vi "ResultsDB Select data_FGV.vi"(6 "Upload Num":string="1", 7 "CMD":T1(ring), 8 "error in (no error)":errorcluster, 9 "ItemsID":string, 11 "MainBarcode":string) -> (0 "error out":errorcluster, 2 "File Paht":string[](array[string]), 3 "30 rows":string[][](array[string]))   [LabVIEW 2021, in "SQLite.lvclass"]
doc: "开始测试时根据条目自动创建条目条目，生产文件路径。\n#2020-6-8 13:25:45"
uses:
  SQLite.lvclass
  <vilib>/Utility/error.llb/Trim Whitespace.vi
  SQLite.lvclass/SQLite.ctl
  <userlib>/LabSQL/LabSQL.lvlib
  vi.lib_New/TopPath/TopPath.lvlib
  <userlib>/sushu/sushu.lvlib
panel:
  in  "error in (no error) 2":errorcluster
  out "32bit integer":i32
  out "size(s)":i32
  out "Update CMD":string
  out "element":string
  out "Table Control":string[][](table)
  out "CMD":string
  out "error out 2":errorcluster
  out "match substring":string
  out "number (0 to 1)":dbl
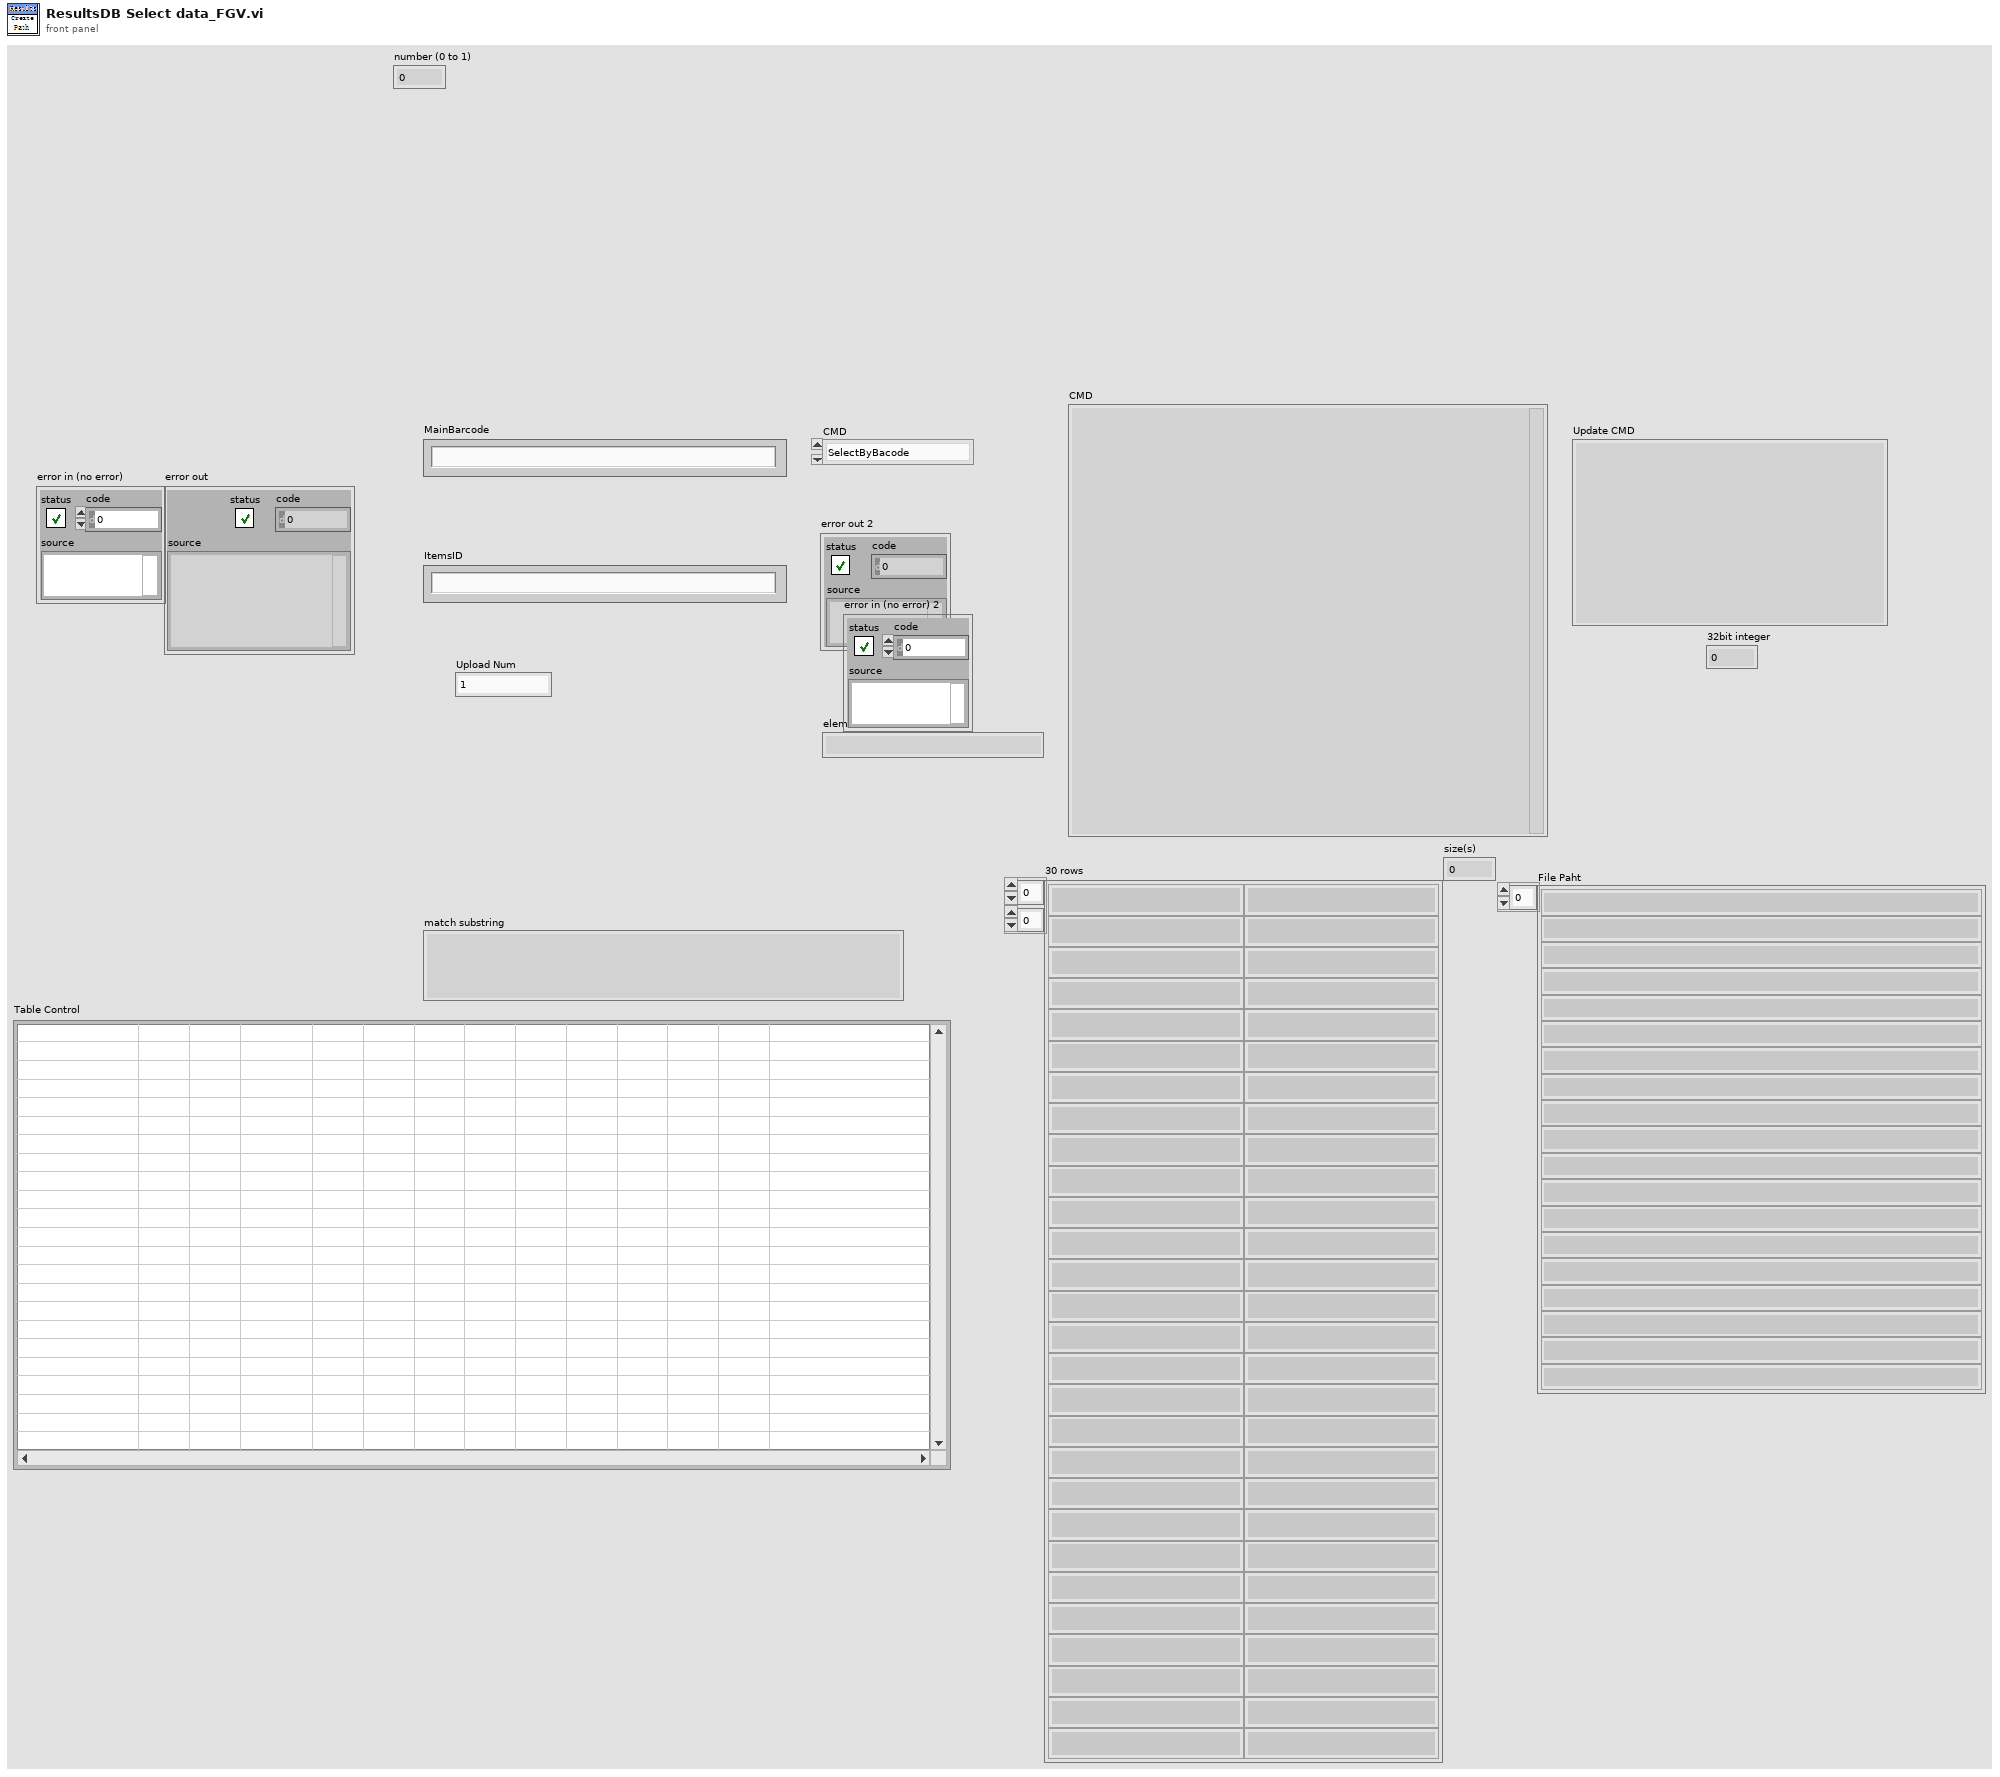
[diagram p1: front panel]
types:
  T1 = enum16{"SelectByBacode", "SelectByDatetime", "Update-UploadColumn"}
  T2 = cluster{"Core":cluster{"Current VI Reference":refnum<vi>, "Close Panel on Exit?":bool}, "VI Name":string, "Row Numbers":string, "Update?":bool, "Results Folder path":path, "CMD":string, "RowNum":i32, "ResultFilePath":path, "InsertTimes":i32, "length":i32}
  T3 = typedef "TopPath.lvlib/Top Path.ctl" = cluster{"LV Source":path, "FilePath":path, "Data":path}
  T4 = enum16{"Other", "SQL2008", "SQLite", "Access", "MySQL"}
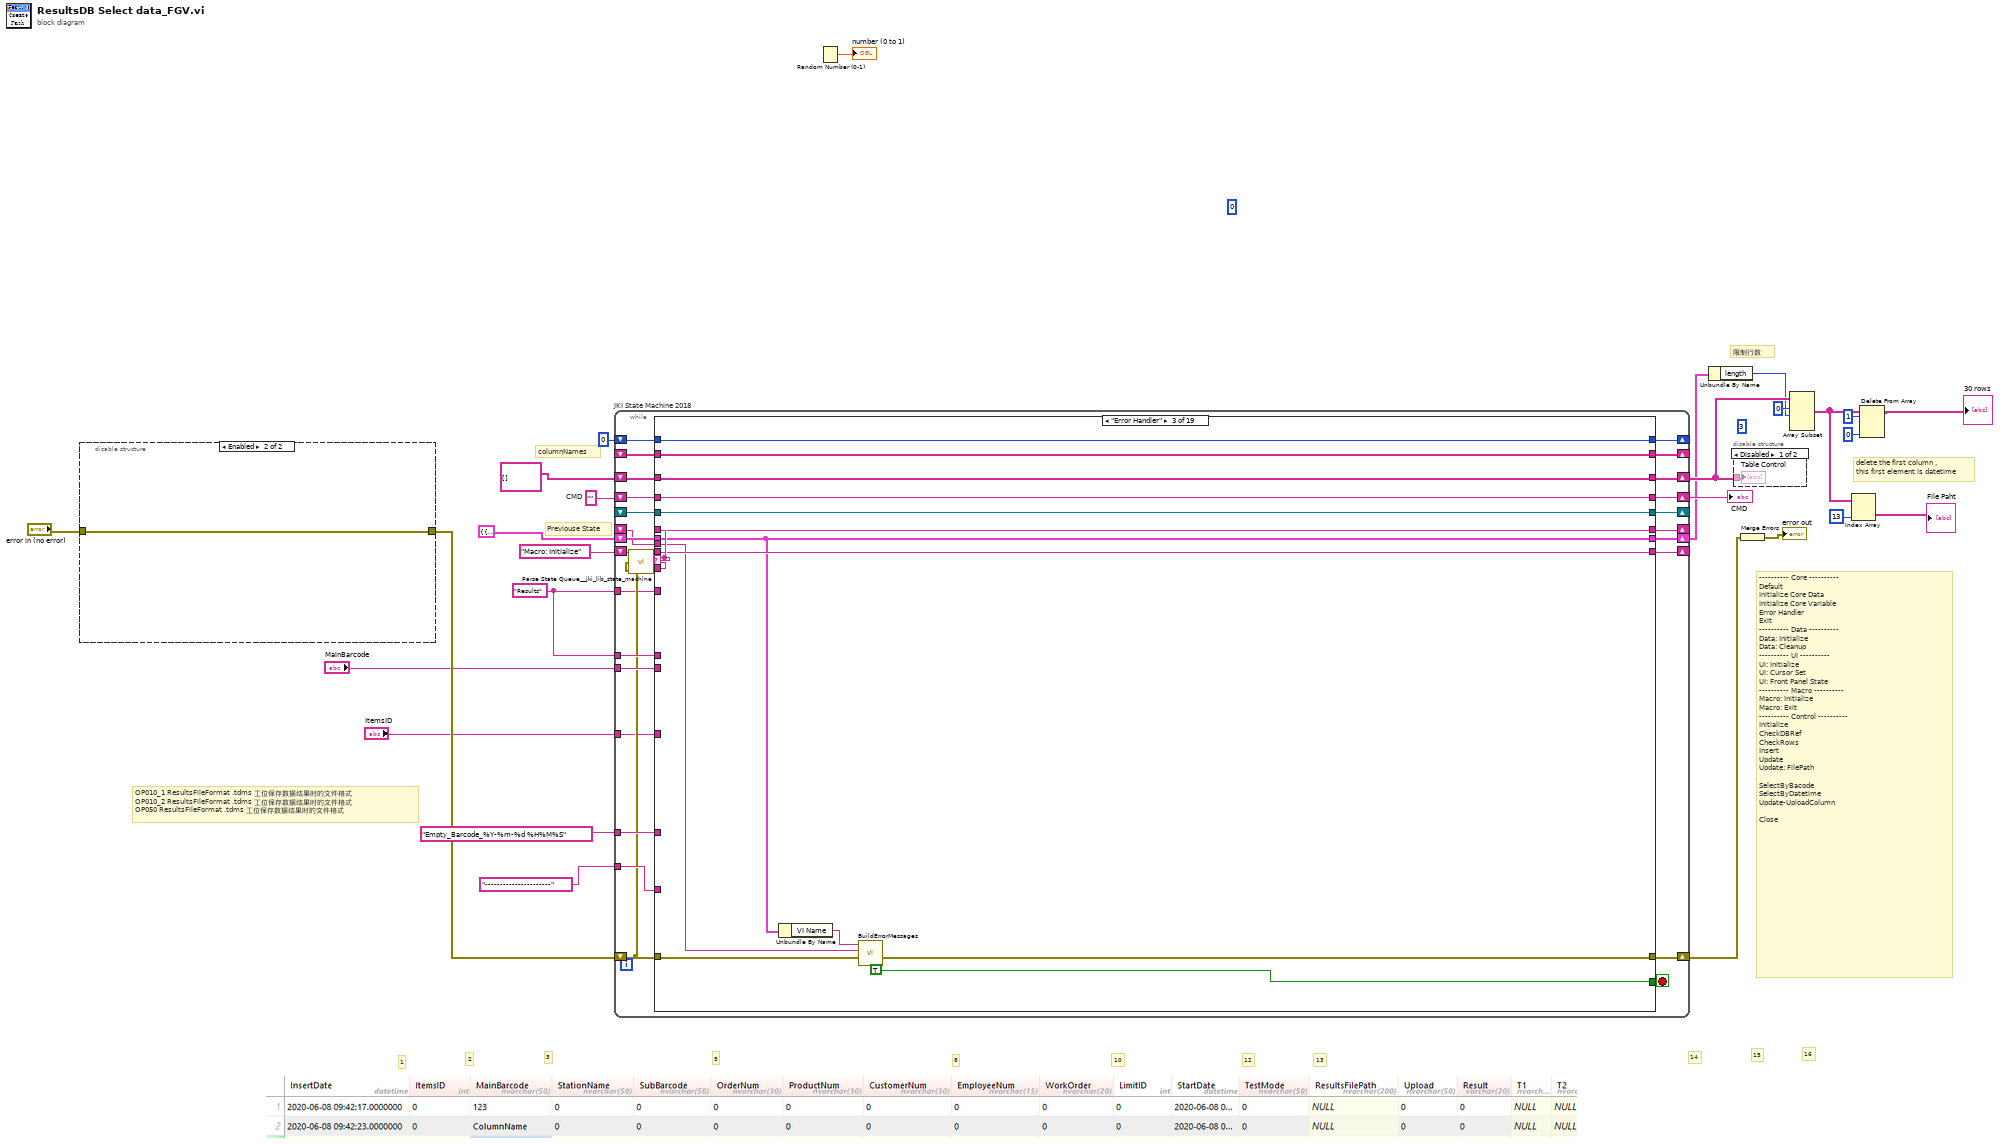
[diagram p0: block diagram]
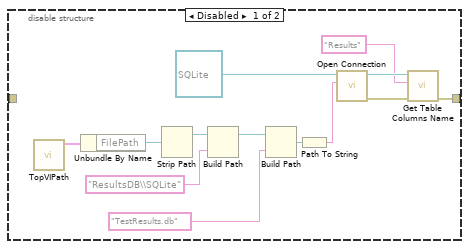
[diagram p2: hidden frame]
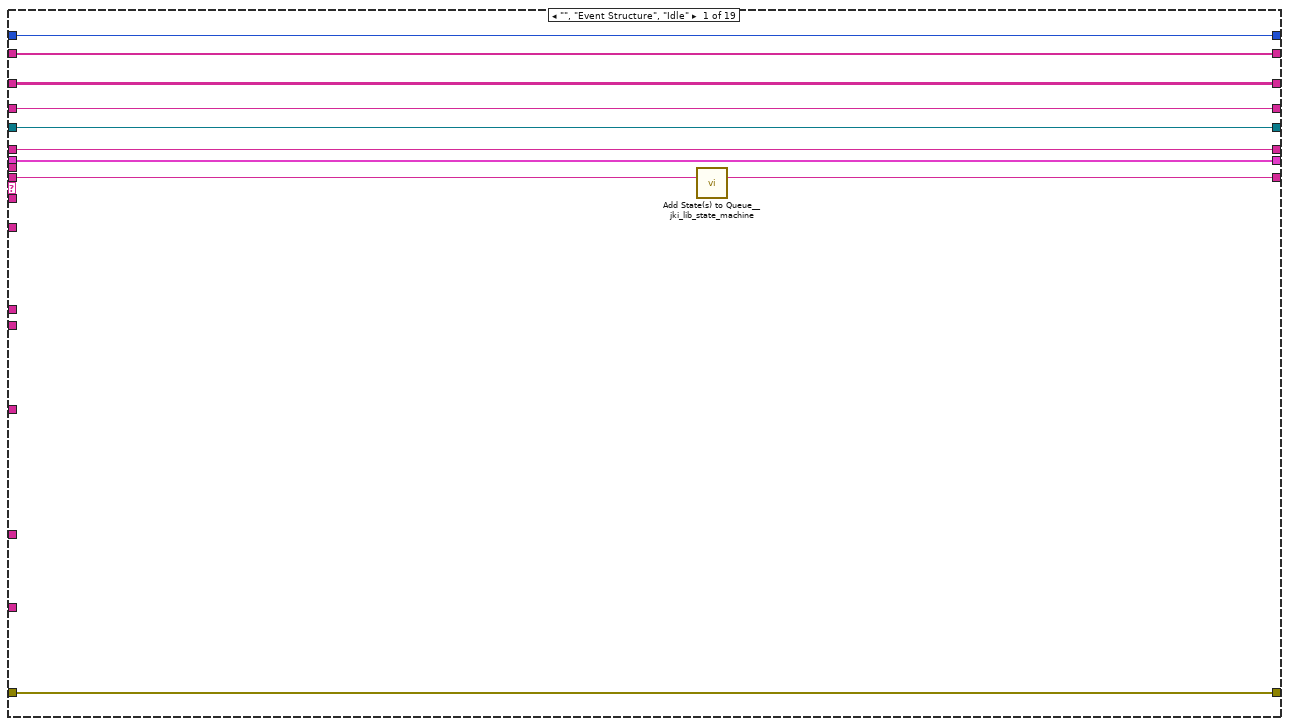
[diagram p4: hidden frame]
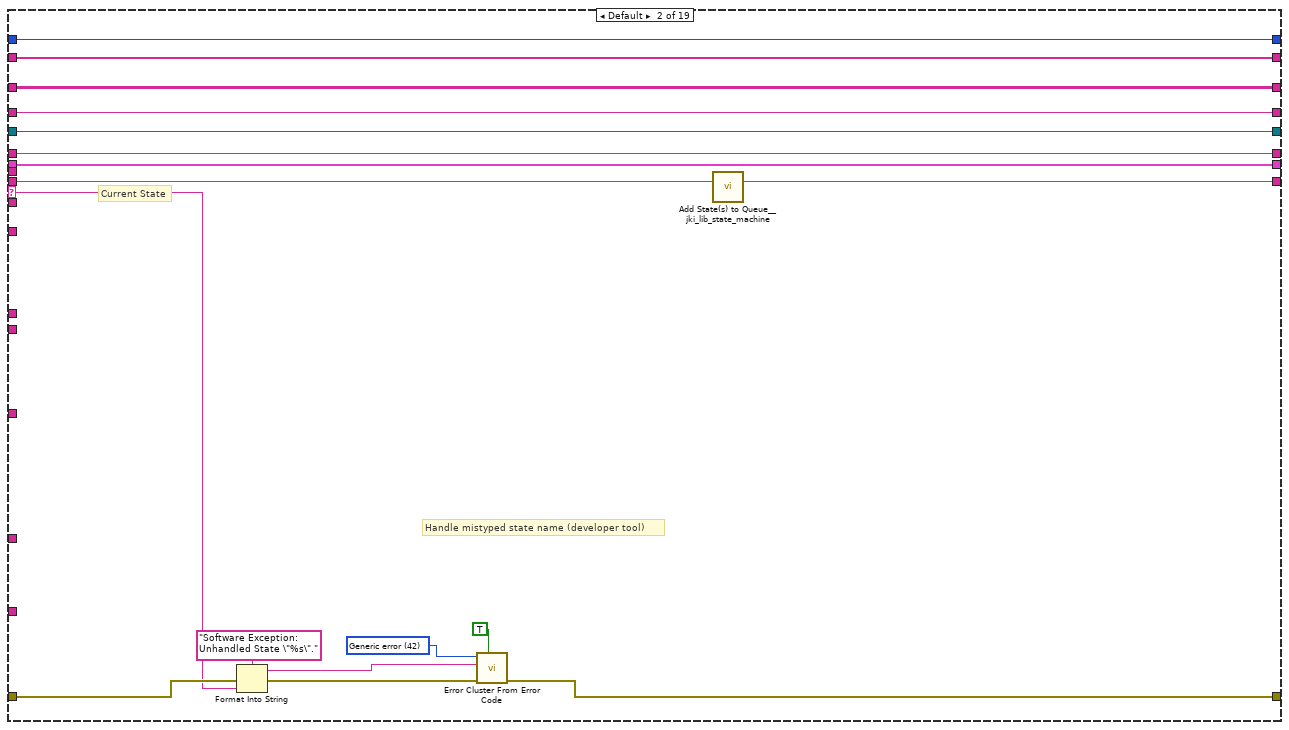
[diagram p5: hidden frame]
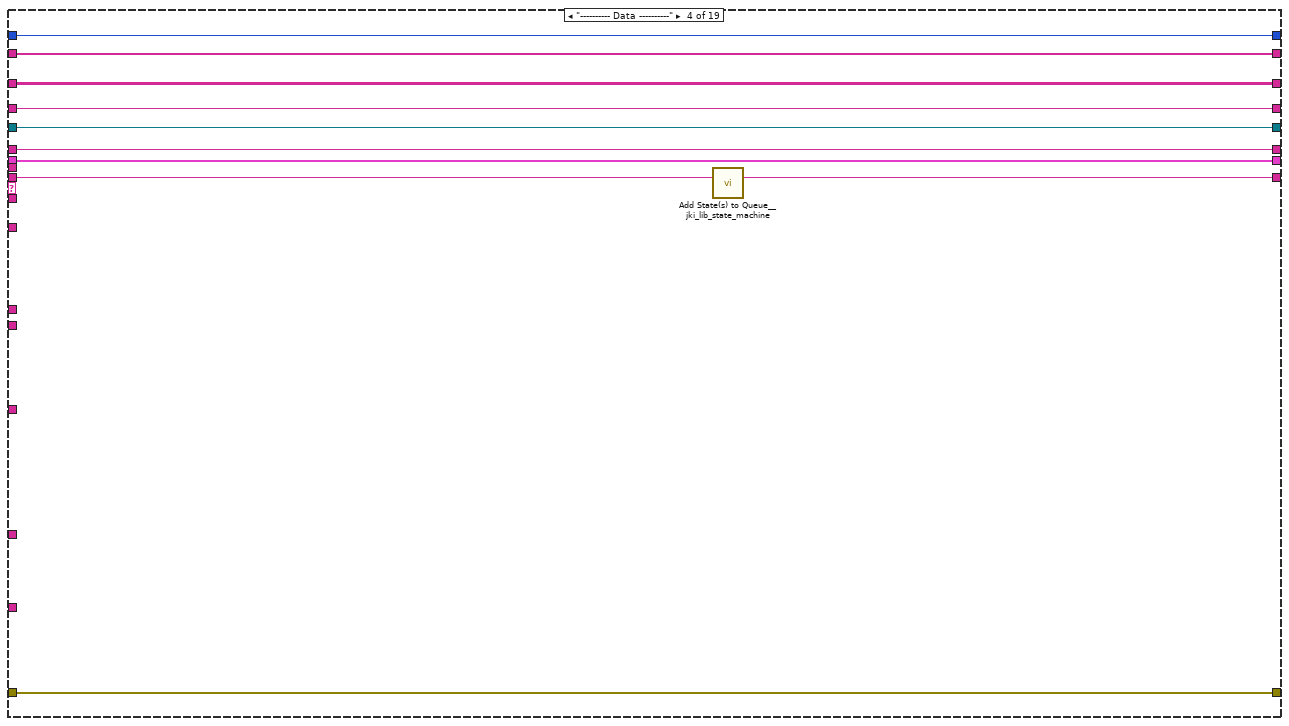
[diagram p6: hidden frame]
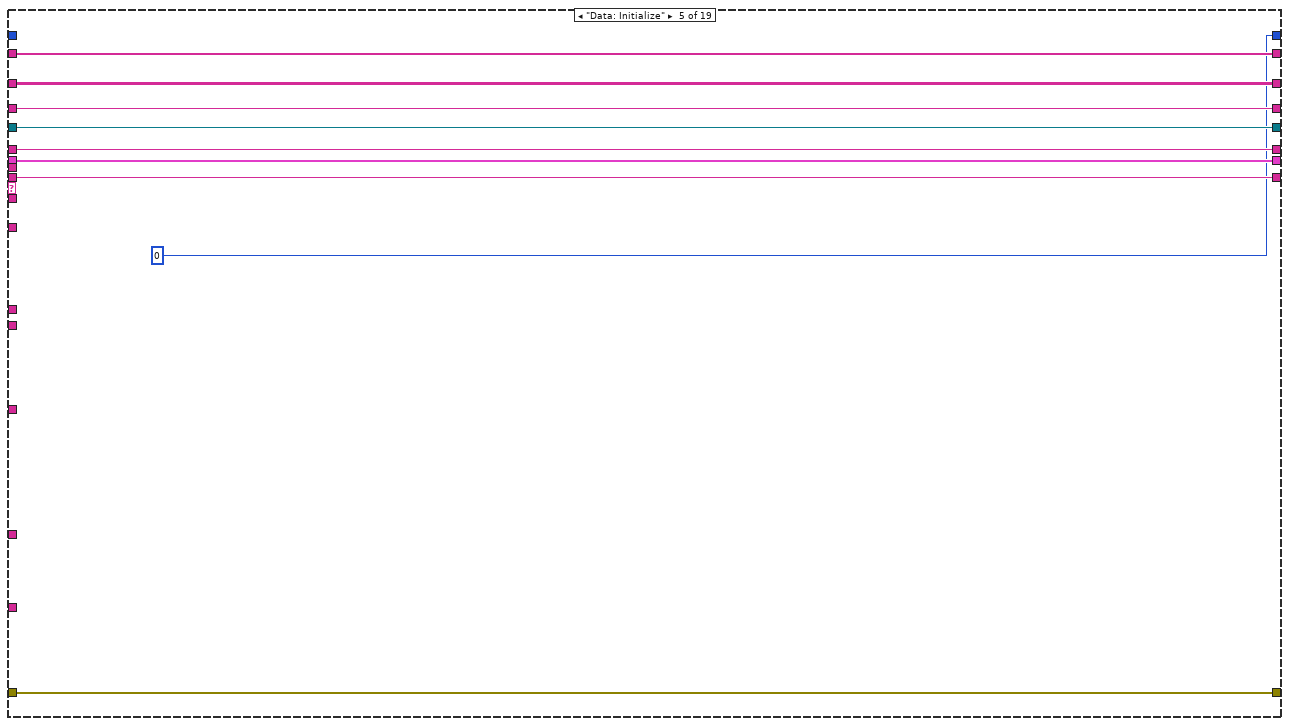
[diagram p7: hidden frame]
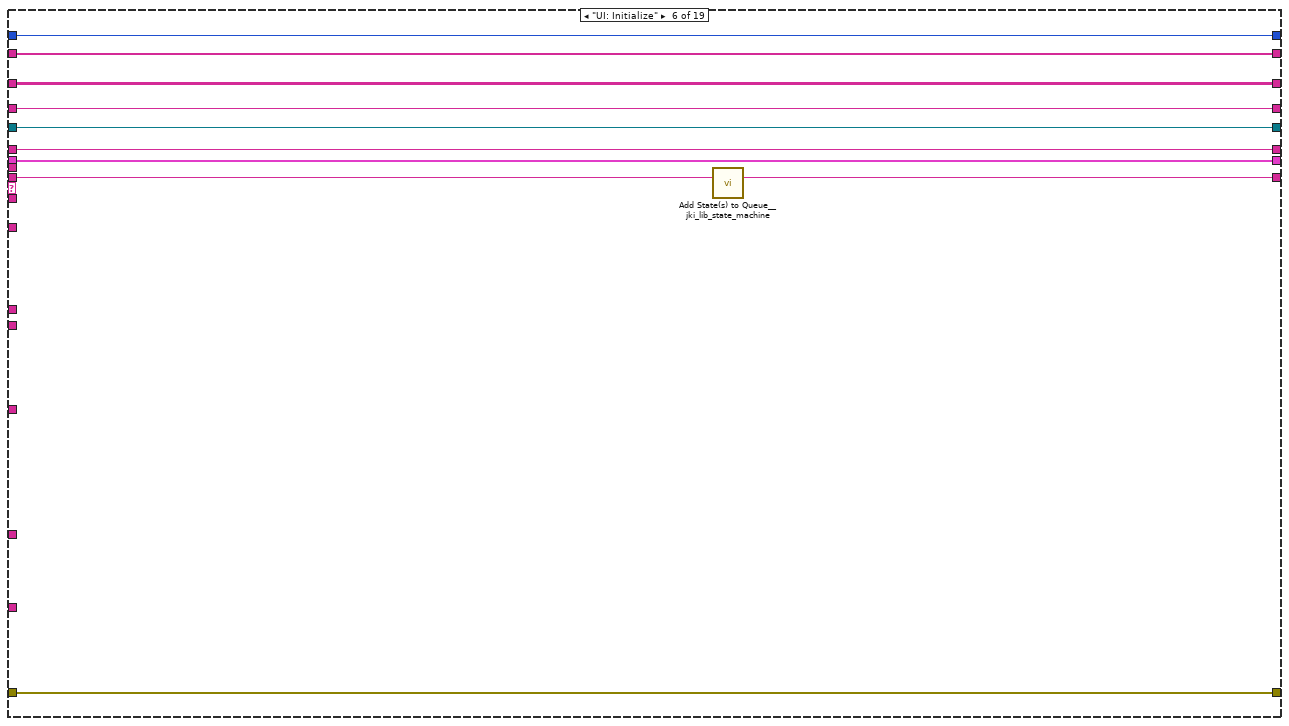
[diagram p8: hidden frame]
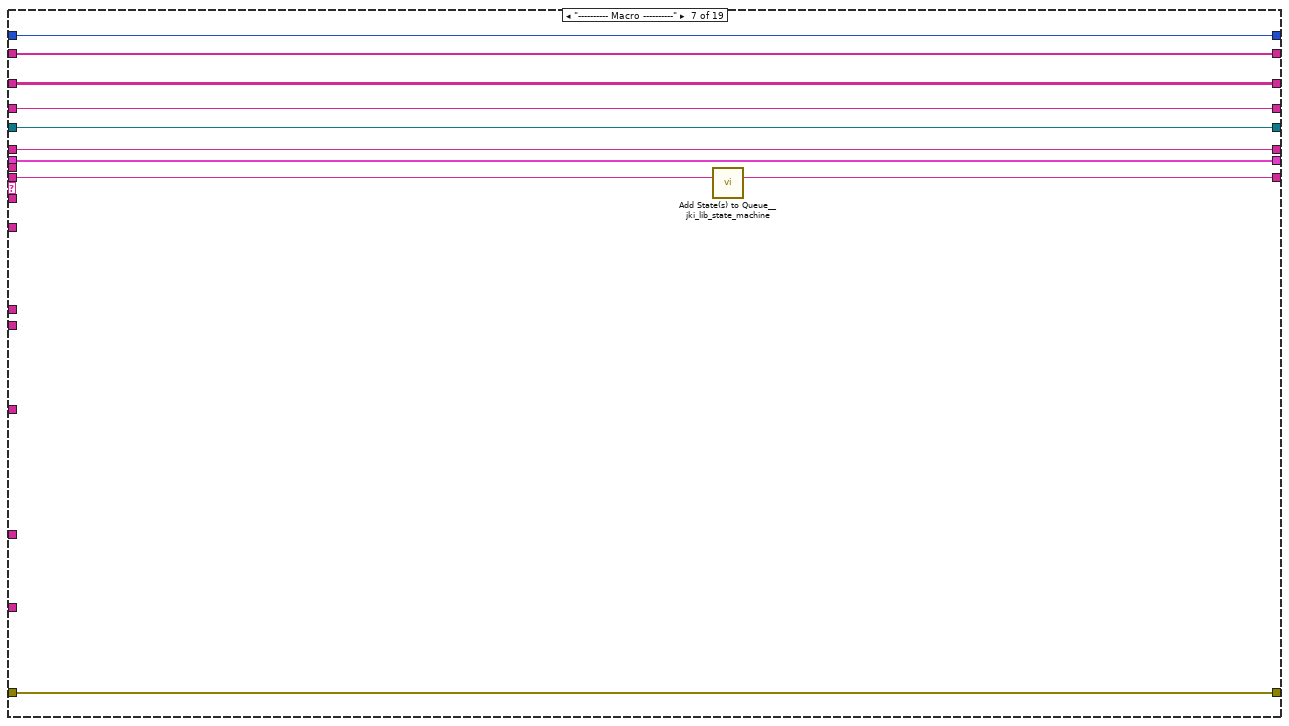
[diagram p9: hidden frame]
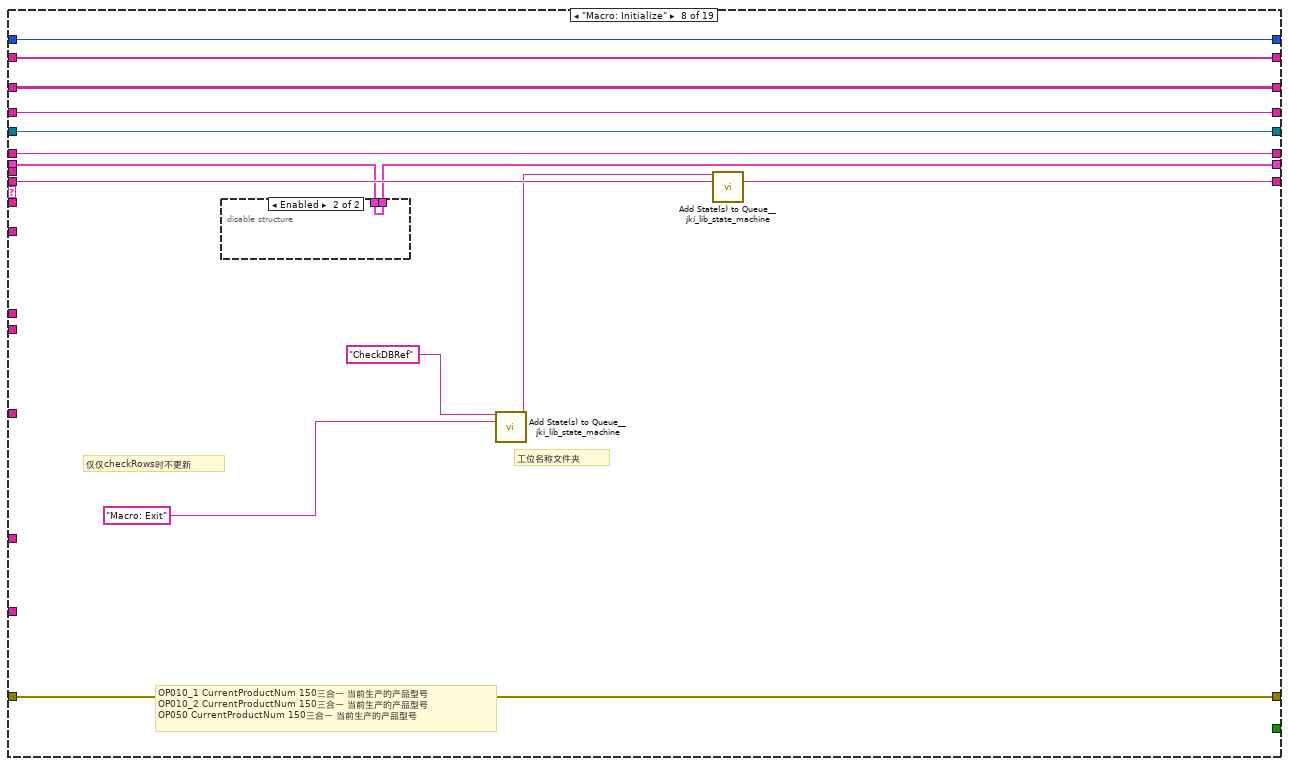
[diagram p10: hidden frame]
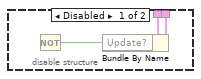
[diagram p11: hidden frame]
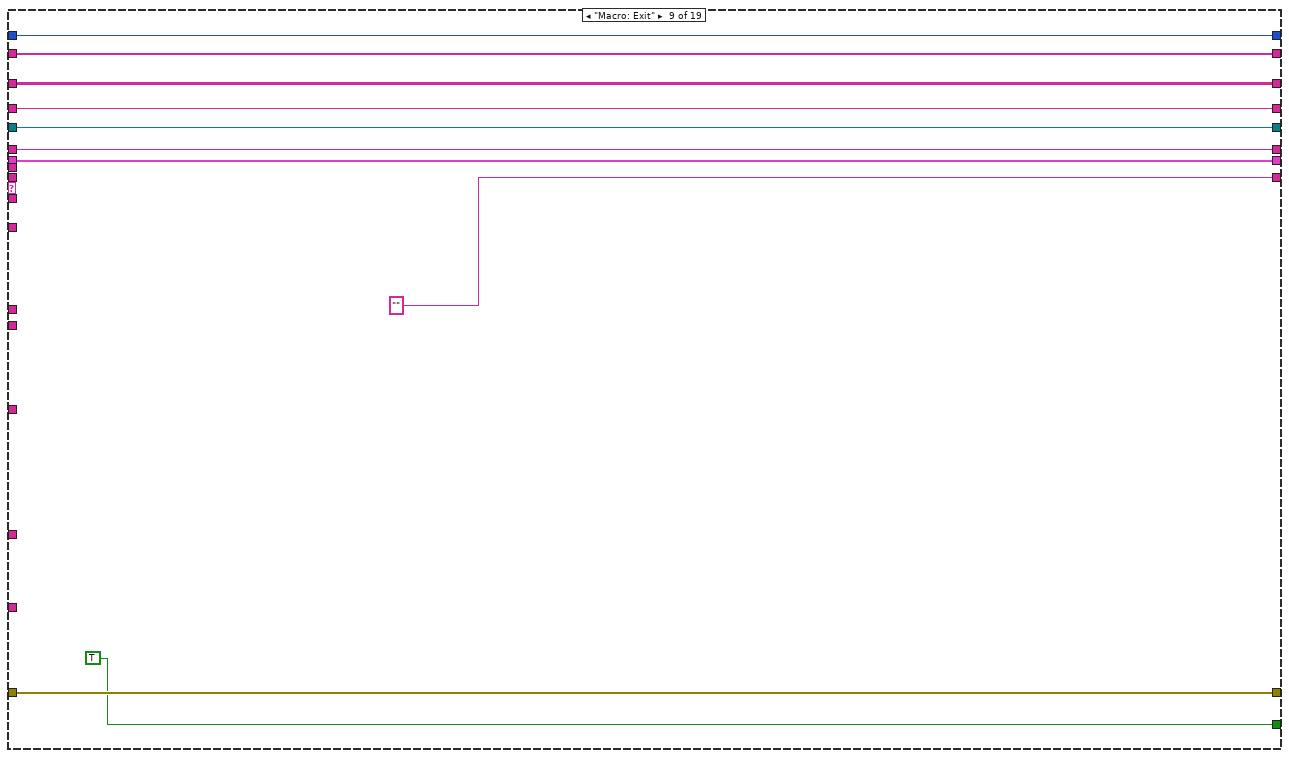
[diagram p12: hidden frame]
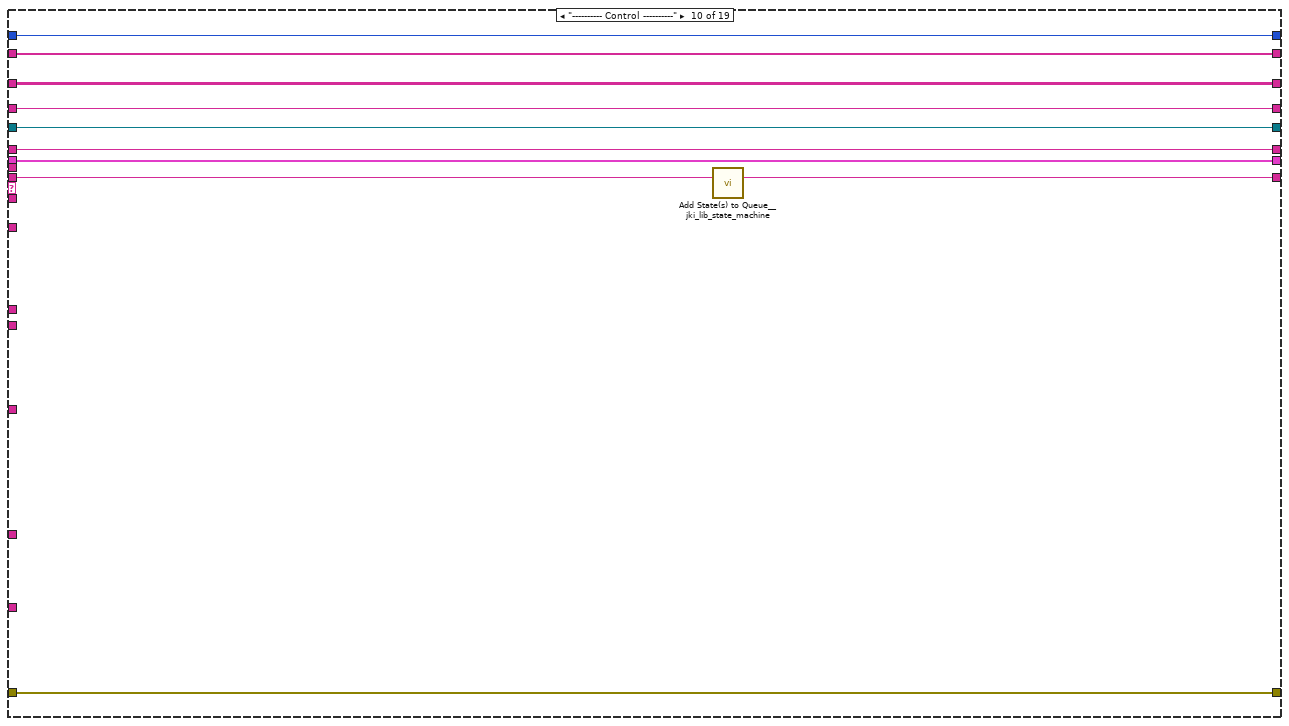
[diagram p13: hidden frame]
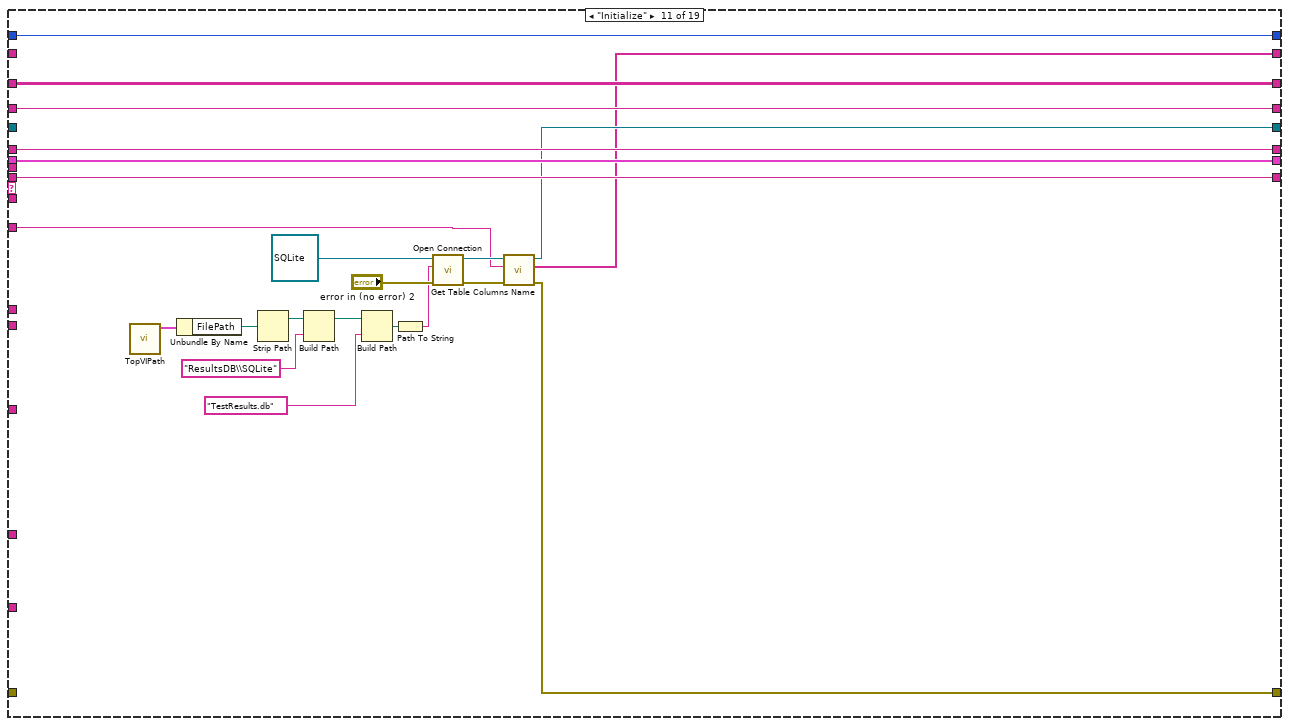
[diagram p14: hidden frame]
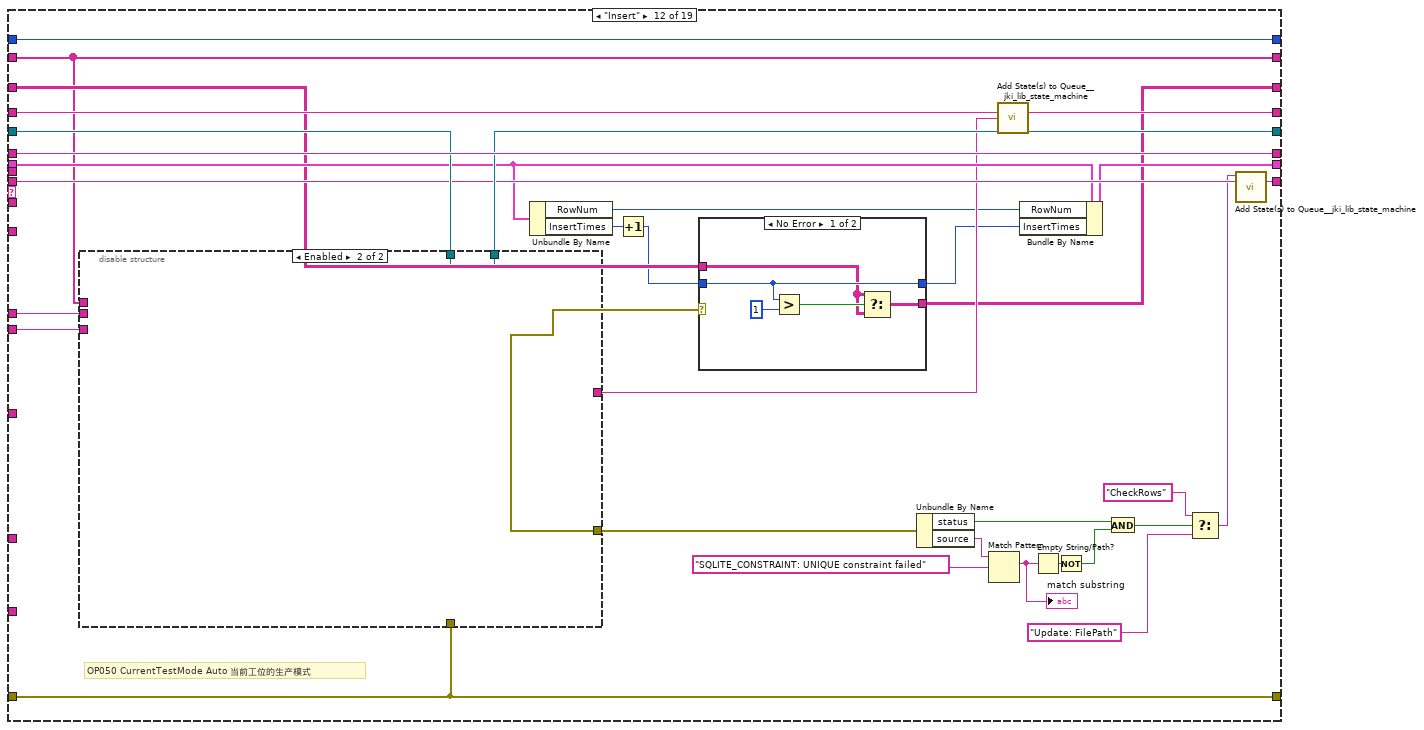
[diagram p15: hidden frame]
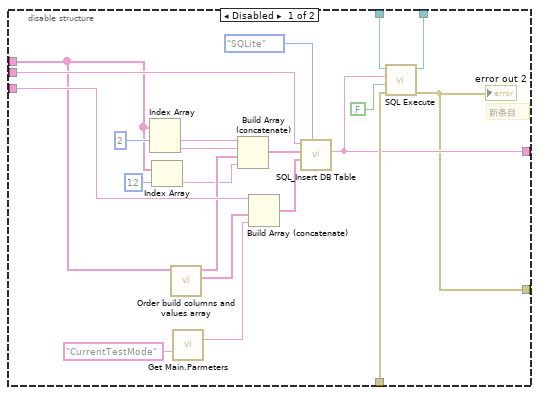
[diagram p16: hidden frame]
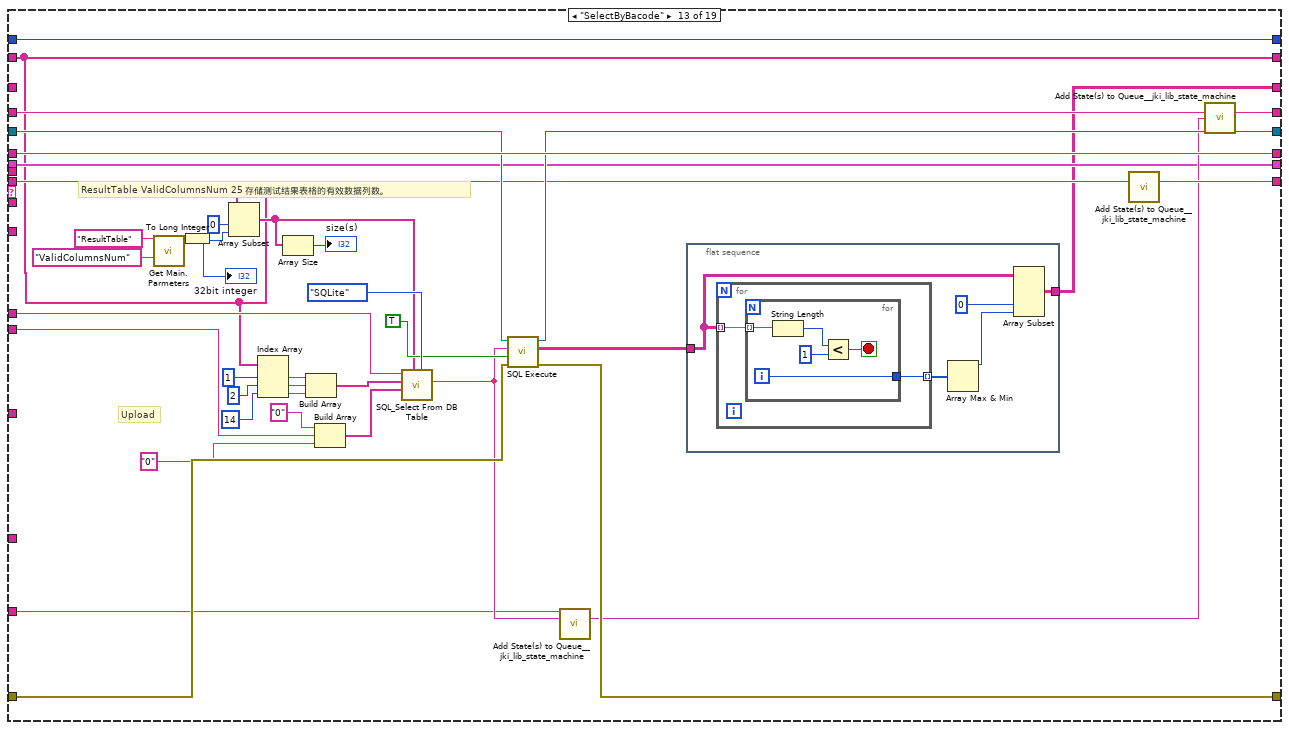
[diagram p18: hidden frame]
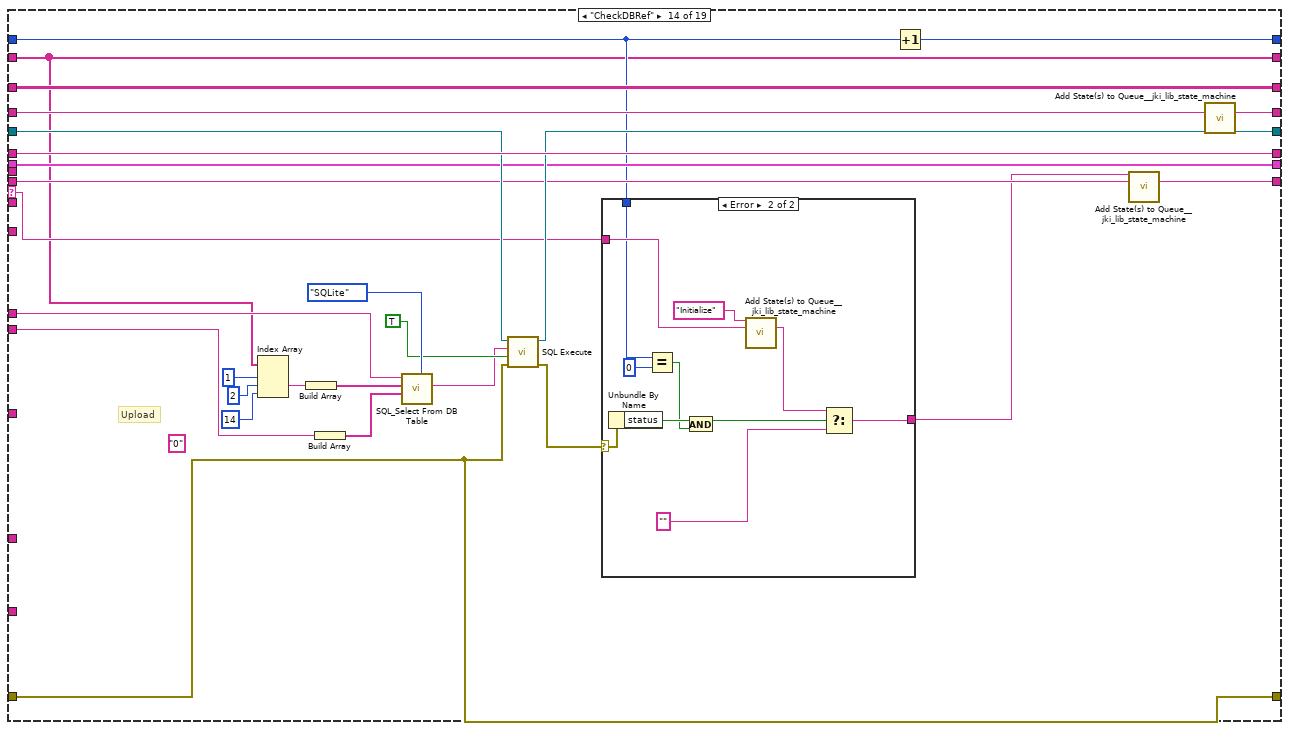
[diagram p19: hidden frame]
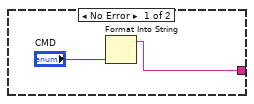
[diagram p20: hidden frame]
diagram:
  w5 = "Results" ("TableName")
  (unwired) 3 ("length")
  w15 = ""  # CMD
  (unwired) 0 ("index (row)")
  # "columnNames"
  # "delete the first column ,\nthis first element is datetime"
  # "限制行数"
  # "OP010_1\tResultsFileFormat\t.tdms\t工位保存数据结果时的文件格式\nOP010_2\tResultsFileFormat\t.tdms\t工位保存数据结果时的文件格式\nOP050\tResultsFileFormat\t.tdms\t工位保存数据结果时的文件格式"
  # "16"
  # "15"
  # "14"
  # "13"
  # "12"
  # "10"
  # "8"
  # "5"
  # "3"
  # "2"
  # "1"
  # "Previouse State"
  # "---------- Core ----------\nDefault\nInitialize Core Data\nInitialize Core Variable\nError Handler\nExit\n---------- Data ----------\nData: Initialize\nData: Cleanup\n---------- UI ----------\nUI: Initialize\nUI: Cursor Set\nUI: Front Panel State\n---------- Macro ----------\nMacro: Initialize\nMacro: Exit\n---------- Control ----------\nInitialize\nCheckDBRef\nCheckRows\nInsert\nUpdate\nUpdate: FilePath\n\nSelectByBacode\nSelectByDatetime\nUpdate-UploadColumn\n\nClose"
  n1 = disable-structure shown="Enabled" {
    disable-tunnel: [w28 w41] -> w21
    disable-tunnel: "error in (no error)" -> [_ w41]
    frame Disabled {
      n2 = call "TopVIPath.vi"() -> ("TopPath"=w29:T3)  [unwired: 10 in, 1 out]
      n3 = Unbundle By Name(w29) -> ("FilePath"=w40:path)
      n4 = Strip Path(path=w40) -> (stripped path=w39:path)  [unwired: 1 out]
      n5 = Build Path(base path=w39, name or relative path="ResultsDB\\SQLite") -> (appended path=w37:path)
      n6 = Build Path(base path=w37, name or relative path="TestResults.db") -> (appended path=w35:path)
      n7 = Path To String(path=w35) -> (string=w34:string)
      n8 = call-dynamic "Open Connection.vi"("ConnectionString"=w34, "HostDB in"=refnum<class "SQLite.lvclass"> refnum ("SQLite.lvclass")) -> ("error out"=w31:errorcluster, "HostDB out"=w32:refnum<class "SQLite.lvclass">, "error in (no error)"=w33:errorcluster)  [unwired: 7 in]
      n9 = call-dynamic "Get Table Columns Name.vi"("error in (no error)"=w31, "TableName"="Results", "HostDB in"=w32) -> ("error out"=w28:errorcluster)  [unwired: 4 in, 4 out]
    }
    frame Enabled {
    }
  }
  n10 = while "JKI State Machine 2018" {
    shift-right: [w63] -> w3
    shift-left: T2 {"Core"={"Current VI Reference"=refnum, "Close Panel on Exit?"=FALSE}, "VI Name"="", "Row Numbers"="", "Update?"=FALSE, "Results Folder path"=path "", "CMD"="", "RowNum"=0, "ResultFilePath"=path "", "InsertTimes"=0, "length"=3} ("Data") -> [w62]
    shift-right: [w66] -> w22
    shift-left: w21 -> [w48]
    shift-right: [w65] -> _
    shift-left: "Macro: Initialize" -> [w67]
    shift-right: [w60] -> _
    shift-left: _ -> [w61]
    shift-right: [w58] -> _
    shift-left: _ -> [w57]
    tunnel: "MainBarcode" -> [w56]
    tunnel: w5 -> [w55]
    tunnel: "Empty_Barcode_%Y-%m-%d %H%M%S" ("time format string (%c)") -> [w54]
    shift-right: [w53] -> w17
    shift-left: w15 -> [w52]
    tunnel: "----------------------" ("State(s) in (\"\")") -> [w51]
    shift-right: [w49] -> w13
    shift-left: string[][] [] ("Table Control") -> [w50]
    tunnel: "ItemsID" -> [w47]
    tunnel: w5 -> [w46]
    shift-right: [w45] -> _
    shift-left: _ -> [w44]
    shift-right: [w42] -> _
    shift-left: 0 -> [w43]
    stop <- w64 stop-if-true
    n11 = call <vilib>:"Parse State Queue__jki_lib_state_machine.vi"("State Queue"=w67, "Error In (no error)"=w48) -> ("Remaining States"=w69:string, "Current State"=w59:string, "Arguments"=w68:string)  [unwired: 10 in, 1 out]
    n12 = case shown="\"Error Handler\"" w59 {
      selector: w59 -> [_ w86 _ _ _ _ _ _ _ _ _ _ _ w325 _ _ _ _ _]
      tunnel: w69 -> [w79 w90 w108 w119 w125 w138 w148 w162 _ w186 w208 w225 w297 w335 w393 w441 w473 w521 w548]
      tunnel: w68 -> [_ _ _ _ _ _ _ _ _ _ _ _ _ _ _ _ _ _ _]
      tunnel: w62 -> [w76 w88 w105 w116 w126 w136 w145 w157 w175 w183 w207 w222 w289 w331 w385 w440 w472 w501 w547]
      tunnel: [w77 w92 w101 w117 w128 w135 w146 w158 w176 w184 w190 w235 w295 w324 w391 w443 w475 w487 w538] -> w66
      tunnel: w48 -> [w77 w91 w102 w117 w128 w135 w146 w158 w176 w184 _ w235 w296 w324 w392 w443 w475 w489 w539]
      tunnel: [w78 w89 w108 w118 w125 w137 w147 w161 "" w185 w208 w226 w298 w336 w394 w442 w474 w522 w548] -> w65
      tunnel: [_ _ TRUE _ _ _ _ _ TRUE _ _ _ _ _ _ _ _ _ _] -> w64
      tunnel: [w76 w88 w105 w116 w126 w136 w145 w152 w175 w183 w207 w221 w289 w331 w361 w440 w472 w494 w547] -> w63
      tunnel: w61 -> [w75 w85 w107 w115 w127 w134 w144 w160 w174 w182 _ w237 w301 w339 w396 w446 w478 w524 w541]
      tunnel: [w75 w85 w107 w115 w127 w134 w144 w160 w174 w182 w191 w236 w300 w338 w395 w445 w477 w523 w540] -> w60
      tunnel: w59 -> [w74 w84 w106 w114 w124 w133 w143 w159 w172 w181 w206 w240 w307 w346 w403 w452 w484 w529 w546]
      tunnel: [w74 w84 w106 w114 w124 w133 w143 w159 w172 w181 w206 w240 w307 w346 w403 w452 w484 w529 w546] -> w58
      tunnel: w57 -> [_ _ w103 _ _ _ _ _ _ _ _ _ _ _ _ _ _ _ _]
      tunnel: w56 -> [_ _ _ _ _ _ _ _ _ _ _ w238 w302 w340 _ w447 w479 w504 _]
      tunnel: w55 -> [_ _ _ _ _ _ _ _ _ _ _ w239 w303 w341 w397 w448 w480 w525 _]
      tunnel: w54 -> [_ _ _ _ _ _ _ _ _ _ _ _ _ _ _ _ _ w503 _]
      tunnel: w52 -> [w73 w83 w100 w113 w123 w132 w142 w154 w170 w180 w205 w220 w293 w333 w389 w422 w461 w499 w545]
      tunnel: [w73 w83 w100 w113 w123 w132 w142 w154 w170 w180 w205 w219 w294 w334 w390 w423 w462 w500 w545] -> w53
      tunnel: w51 -> [_ _ _ _ _ _ _ _ _ _ _ _ w290 _ w386 w419 w458 w496 _]
      tunnel: w50 -> [w72 w82 w99 w112 w122 w131 w141 w153 w169 w179 w204 w215 _ w327 _ w418 w457 w488 w544]
      tunnel: [w72 w82 w99 w112 w122 w131 w141 w153 w169 w179 w204 w214 w284 w327 w364 w418 w457 w488 w544] -> w49
      tunnel: w47 -> [_ _ _ _ _ _ _ _ _ _ _ _ _ _ _ _ w455 _ _]
      tunnel: w46 -> [_ _ _ _ _ _ _ _ _ _ w189 _ _ _ _ _ _ _ _]
      tunnel: w44 -> [w71 w81 w98 w111 w121 w130 w140 w151 w168 w178 _ w209 w272 w320 w362 w416 w453 w485 w543]
      tunnel: [w71 w81 w98 w111 w121 w130 w140 w151 w168 w178 w188 w209 w272 w320 w362 w416 w453 w485 w543] -> w45
      tunnel: w43 -> [w70 w80 w97 w110 _ w129 w139 w149 w167 w177 w187 w210 w273 w321 w363 w417 w454 w486 w542]
      tunnel: [w70 w80 w97 w110 0 w129 w139 w149 w167 w177 w187 w210 w273 w322 w363 w417 w454 w486 w542] -> w42
      frame "", "Event Structure", "Idle" {
        n13 = call <vilib>:"Add State(s) to Queue__jki_lib_state_machine.vi"("State(s) in (\"\")"=w79) -> ("States Out"=w78:string)  [unwired: 14 in]
      }
      frame Default {
        w95 = 42 items=["No error", "Argument error", "Memory is full", "Out of zone", "End of file", "File already open", "Generic file I/O error", "File not found", "File permission error", "Disk is full", "Duplicate path", "Too many files open", "System feature not enabled", "Resource file not found", "Cannot add resource", "Resource not found", "Image not found", "Image memory error", "Pen does not exist", "Config type invalid", "Config token not found", "Config parse error", "Config memory error", "Bad external code format", "Bad external code offset", "External code not present", "Null window", "Destroy window error", "Null menu", "Print aborted", "Bad print record", "Print driver error", "Windows error during printing", "Memory error during printing", "Print dialog error", "Generic print error", "Invalid device refnum", "Device not found", "Device parameter error", "Device unit error", "Cannot open device", "Device call aborted", "Generic error", "Cancelled by user", "Object ID too low", "Object ID too high", "Object not in heap", "Unknown heap", "Unknown object (invalid DefProc)", "Unknown object (DefProc not in table)", "Message out of range", "Invalid (null) method", "Unknown message", "Manager call not supported", "Bad address", "Network operation in progress", "Network operation timed out", "Connection is busy", "Network attribute not supported", "Network error", "Address in use", "System out of memory", "Connection aborted", "Connection refused", "Not connected", "Already connected", "Connection closed", "Initialization error (interapplication manager)", "Bad occurrence", "Wait on unbound occurrence handler", "Occurrence queue overflow", "Datalog type conflict", "Unused", "Unrecognized type (interapplication manager)", "Memory corrupt", "Failed to make temporary DLL", "Old CIN version", "Drag socket not found", "Failed to load drop-object", "Failed to register OLE object", "Failed to release OLE object", "Format specifier type mismatch", "Unknown format specifier", "Too few format specifiers", "Too many format specifiers", "Scan failed", "Newer CIN version", "Error converting to variant", "Runtime menu error", "Password tampered", "Variant attribute not found", "Incompatible variant data type", "Event data is not available", "Event Store is not present", "Occurrence is not found", "Event Queue is not created", "Event info is not available", "Refnum passed is NULL", "Error retrieving Class GUID", "Error retrieving CoClass GUID", "Error retrieving TypeLib GUID.", "Bad built application magic bytes.", "Specific driver is different from the specific driver associated with the Logical Name.", "There is no session opened to the class driver.", "Max Error", "MAX - Error with config objects", "MAX - Error loading configuration", "MAX - Group not supported"]
        # "Current State"
        # "Handle mistyped state name (developer tool)"
        n14 = Format Into String(format string="Software Exception: Unhandled State \"%s\"." ("message"), error in=w91, w86) -> (resulting string=w94:string, error out=w93:errorcluster)  [unwired: 1 in]
        n15 = call <vilib>:"Error Cluster From Error Code.vi"("show call chain? (False)"=TRUE, "error in (no error)"=w93, "error message (\"\")"=w94, "error code (0)"=w95) -> ("error out"=w92:errorcluster)  [unwired: 5 in]
        n16 = call <vilib>:"Add State(s) to Queue__jki_lib_state_machine.vi"("State(s) in (\"\")"=w90) -> ("States Out"=w89:string)  [unwired: 14 in]
      }
      frame "Error Handler" {
        n17 = Unbundle By Name(w105) -> ("VI Name"=w104:string)
        n18 = call <userlib>:"BuildErrorMessages.vi"("error in"=w102, "ErrorCase"=w103, "VI Name"=w104) -> ("error out (no error)"=w101:errorcluster)  [unwired: 6 in, 2 out]
      }
      frame "---------- Data ----------" {
        n19 = call <vilib>:"Add State(s) to Queue__jki_lib_state_machine.vi"("State(s) in (\"\")"=w119) -> ("States Out"=w118:string)  [unwired: 14 in]
      }
      frame "Data: Initialize" {
      }
      frame "UI: Initialize" {
        n20 = call <vilib>:"Add State(s) to Queue__jki_lib_state_machine.vi"("State(s) in (\"\")"=w138) -> ("States Out"=w137:string)  [unwired: 14 in]
      }
      frame "---------- Macro ----------" {
        n21 = call <vilib>:"Add State(s) to Queue__jki_lib_state_machine.vi"("State(s) in (\"\")"=w148) -> ("States Out"=w147:string)  [unwired: 14 in]
      }
      frame "Macro: Initialize" {
        # "OP010_1\tCurrentProductNum\t150三合一\t当前生产的产品型号\nOP010_2\tCurrentProductNum\t150三合一\t当前生产的产品型号\nOP050\tCurrentProductNum\t150三合一\t当前生产的产品型号"
        # "工位名称文件夹"
        # "仅仅checkRows时不更新"
        n22 = disable-structure shown="Enabled" {
          disable-tunnel: w157 -> [w165 w166]
          disable-tunnel: [w164 w166] -> w152
          frame Disabled {
            n23 = Not() -> (.not. x?=w163:bool)  [unwired: 1 in]
            n24 = Bundle By Name(cluster=w165, "Update?"=w163) -> (w164:T2)
          }
          frame Enabled {
          }
        }
        n25 = call <vilib>:"Add State(s) to Queue__jki_lib_state_machine.vi"("State(s) in Front (\"\")"="CheckDBRef" ("State(s) in Front (\"\")"), "State(s) in (\"\")"="Macro: Exit") -> ("States Out"=w156:string)  [unwired: 13 in]
        n26 = call <vilib>:"Add State(s) to Queue__jki_lib_state_machine.vi"("State(s) in Front (\"\")"=w156, "State(s) in (\"\")"=w162) -> ("States Out"=w161:string)  [unwired: 13 in]
      }
      frame "Macro: Exit" {
      }
      frame "---------- Control ----------" {
        n27 = call <vilib>:"Add State(s) to Queue__jki_lib_state_machine.vi"("State(s) in (\"\")"=w186) -> ("States Out"=w185:string)  [unwired: 14 in]
      }
      frame "Initialize" {
        n28 = call "TopVIPath.vi"() -> ("TopPath"=w203:T3)  [unwired: 10 in, 1 out]
        n29 = Unbundle By Name(w203) -> ("FilePath"=w192:path)
        n30 = Strip Path(path=w192) -> (stripped path=w193:path)  [unwired: 1 out]
        n31 = Build Path(base path=w193, name or relative path="ResultsDB\\SQLite") -> (appended path=w195:path)
        n32 = Build Path(base path=w195, name or relative path="TestResults.db") -> (appended path=w197:path)
        n33 = Path To String(path=w197) -> (string=w198:string)
        n34 = call-dynamic "Open Connection.vi"("error in (no error)"="error in (no error) 2", "ConnectionString"=w198, "HostDB in"=refnum<class "SQLite.lvclass"> refnum ("SQLite.lvclass")) -> ("error out"=w201:errorcluster, "HostDB out"=w200:refnum<class "SQLite.lvclass">)  [unwired: 7 in]
        n35 = call-dynamic "Get Table Columns Name.vi"("error in (no error)"=w201, "TableName"=w189, "HostDB in"=w200) -> ("error out"=w190:errorcluster, "Table_ColunmsList"=w188:string[], "HostDB out"=w191:refnum<class "SQLite.lvclass">)  [unwired: 4 in, 2 out]
      }
      frame "Insert" {
        # "OP050\tCurrentTestMode\tAuto\t当前工位的生产模式"
        n36 = disable-structure shown="Enabled" {
          disable-tunnel: w239 -> [w255 _]
          disable-tunnel: w238 -> [w254 _]
          disable-tunnel: w237 -> [w253 w262]
          disable-tunnel: [w252 w262] -> w236
          disable-tunnel: w235 -> [w250 _]
          disable-tunnel: [w247 _] -> w218
          disable-tunnel: w209 -> [w244 _]
          disable-tunnel: [w241 _] -> w216
          frame Disabled {
            # "新条目"
            n37 = Index Array(array=w244, index #1=2 ("index")) -> (element #1=w260:string, element #2=w261:string)  [unwired: 1 in]
            n38 = Index Array(array=w244, index=12) -> (element=w242:string)
            n39 = call "Order build columns and values array.vi"("ColunmsList"=w244) -> ("Order values Array"=w248:string[], "Order Columns Array"=w249:string[])  [unwired: 9 in]
            n40 = call "Get Main.Parmeters.vi"("VariableName"="CurrentTestMode") -> ("Value"=w245:string)  [unwired: 7 in, 7 out]
            n41 = Build Array (concatenate)(w260, w261, w249, w242) -> (w258:string[])
            n42 = Build Array (concatenate)(w254, w248, w245) -> (w257:string[])  [unwired: 1 in]
            n43 = call <userlib>:"SQL_Insert DB Table.vi"("DB Type"=T4."SQLite", "ColumnsValue"=w257, "ColumnsName"=w258, "Table Name"=w255) -> ("Insert DB String"=w247:string)  [unwired: 7 in]
            n44 = call-dynamic "SQL Execute.vi"("error in (no error)"=w250, "Return Data (T)"=FALSE, "Command Text"=w247, "HostDB in"=w253) -> ("error out"=w241:errorcluster, "HostDB out"=w252:refnum<class "SQLite.lvclass">)  [unwired: 3 in, 3 out]
            "error out 2" <- w241
          }
          frame Enabled {
          }
        }
        n45 = Unbundle By Name(w222) -> ("RowNum"=w217:i32, "InsertTimes"=w212:i32)
        n46 = Increment(x=w212) -> (x+1=w211:i32)
        n47 = case shown="No Error" w216 {
          tunnel: w211 -> [w264 w268]
          tunnel: w215 -> [w263 w269]
          tunnel: [w265 w269] -> w214
          tunnel: [w264 w268] -> w213
          frame No Error {
            n48 = Greater?(x=w264, y=1) -> (0:w266:bool)
            n49 = Select(t=w263, s=w266, f=w263) -> (s? t:f=w265:string[][])
          }
          frame Error {
          }
        }
        n50 = Unbundle By Name(w216) -> ("status"=w231:bool, "source"=w234:string)
        n51 = Match Pattern(string=w234, regular expression="SQLITE_CONSTRAINT: UNIQUE constraint failed") -> (match substring=w232:string)  [unwired: 1 in, 3 out]
        "match substring" <- w232
        n52 = call <vilib>:"Add State(s) to Queue__jki_lib_state_machine.vi"("State(s) in (\"\")"=w220, "State(s) at Back (\"\")"=w218) -> ("States Out"=w219:string)  [unwired: 13 in]
        n53 = Bundle By Name(cluster=w222, "RowNum"=w217, "InsertTimes"=w213) -> (w221:T2)
        n54 = Empty String/Path?(string/path=w232) -> (empty?=w230:bool)
        n55 = Not(x=w230) -> (.not. x?=w223:bool)
        n56 = And(x=w231, y=w223) -> (x .and. y?=w229:bool)
        n57 = Select(t="CheckRows", s=w229, f="Update: FilePath") -> (s? t:f=w224:string)
        n58 = call <vilib>:"Add State(s) to Queue__jki_lib_state_machine.vi"("State(s) in Front (\"\")"=w224, "State(s) in (\"\")"=w225) -> ("States Out"=w226:string)  [unwired: 13 in]
      }
      frame "SelectByBacode" {
        # "ResultTable\tValidColumnsNum\t25\t存储测试结果表格的有效数据列数。"
        # "Upload"
        n59 = call "Get Main.Parmeters.vi"("Main"="ResultTable", "VariableName"="ValidColumnsNum") -> ("DBL Value"=w280:dbl)  [unwired: 6 in, 7 out]
        n60 = To Long Integer(number=w280) -> (32bit integer=w279:i32)
        "32bit integer" <- w279
        n61 = Array Subset(array=w272, index=0, length=w279) -> (w275:string[])
        n62 = Index Array(array=w272, index #1=1 ("index"), index #2=2 ("index"), index #3=14 ("index")) -> (element #1=w271:string, element #2=w287:string, element #3=w277:string)
        n63 = Array Size(array=w275) -> (size(s)=→"size(s)":i32)
        n64 = Build Array(w271, w287, w277) -> (w306:string[])
        n65 = Build Array("0" ("element"), w302, "0" ("State(s) in (\"\")")) -> (w305:string[])
        n66 = call <userlib>:"SQL_Select From DB Table.vi"("DB Type"=T4."SQLite", "SelectedColumnsNameList"=w275, "ColumnsValue"=w305, "ColumnsNameList"=w306, "TableName"=w303) -> ("Select SQL CMD"=w291:string)  [unwired: 6 in]
        n67 = call-dynamic "SQL Execute.vi"("error in (no error)"=w296, "Return Data (T)"=TRUE, "Command Text"=w291, "HostDB in"=w301) -> ("error out"=w295:errorcluster, "Table Control"=w285:string[][], "HostDB out"=w300:refnum<class "SQLite.lvclass">)  [unwired: 3 in, 2 out]
        n68 = call <vilib>:"Add State(s) to Queue__jki_lib_state_machine.vi"("State(s) in Front (\"\")"=w290, "State(s) in (\"\")"=w291) -> ("States Out"=w292:string)  [unwired: 13 in]
        n69 = flat-sequence {
          tunnel: w285 -> [w309]
          tunnel: [w308] -> w284
          frame #0 {
            n70 = for {
              tunnel: w309 -> [w314] mode=indexing
              tunnel: [w313] -> w312 mode=indexing
              n71 = for {
                tunnel: w314 -> [w319] mode=indexing
                tunnel: [w315] -> w313
                i -> [w315]
                stop <- w316 stop-if-true
                n72 = String Length(string=w319) -> (length=w318:i32)
                n73 = Less?(x=w318, y=1) -> (x < y?=w316:bool)
              }
            }
            n74 = Array Max & Min(array=w312) -> (max value=w310:i32)  [unwired: 3 out]
            n75 = Array Subset(array=w309, index (col)=0 ("index"), length (col)=w310) -> (w308:string[][])  [unwired: 2 in]
          }
        }
        n76 = call <vilib>:"Add State(s) to Queue__jki_lib_state_machine.vi"("State(s) in (\"\")"=w297) -> ("States Out"=w298:string)  [unwired: 14 in]
        n77 = call <vilib>:"Add State(s) to Queue__jki_lib_state_machine.vi"("State(s) in (\"\")"=w293, "State(s) at Back (\"\")"=w292) -> ("States Out"=w294:string)  [unwired: 13 in]
      }
      frame "CheckDBRef" {
        (unwired) "0" ("State(s) in (\"\")")
        # "Upload"
        n78 = Index Array(array=w320, index #1=1 ("index"), index #2=2 ("index"), index #3=14 ("index")) -> (element #2=w329:string)  [unwired: 2 out]
        n79 = Build Array(w329) -> (w344:string[])
        n80 = Build Array(w340) -> (w343:string[])
        n81 = call <userlib>:"SQL_Select From DB Table.vi"("DB Type"=T4."SQLite", "ColumnsValue"=w343, "ColumnsNameList"=w344, "TableName"=w341) -> ("Select SQL CMD"=w332:string)  [unwired: 7 in]
        n82 = call-dynamic "SQL Execute.vi"("error in (no error)"=w324, "Return Data (T)"=TRUE, "Command Text"=w332, "HostDB in"=w339) -> ("error out"=w326:errorcluster, "HostDB out"=w338:refnum<class "SQLite.lvclass">)  [unwired: 3 in, 3 out]
        n83 = case shown="Error" w326 {
          selector: w326 -> [_ w355]
          tunnel: w325 -> [_ w356]
          tunnel: [w347 w354] -> w323
          tunnel: w321 -> [_ w351]
          frame No Error {
            n84 = Format Into String("CMD") -> (resulting string=w347:string)  [unwired: 3 in, 1 out]
          }
          frame Error {
            n85 = Unbundle By Name(w355) -> ("status"=w353:bool)
            n86 = Equal?(x=w351, y=0) -> (x = y?=w349:bool)
            n87 = And(x=w353, y=w349) -> (x .and. y?=w352:bool)
            n88 = call <vilib>:"Add State(s) to Queue__jki_lib_state_machine.vi"("State(s) in Front (\"\")"="Initialize" ("Remaining States"), "State(s) in (\"\")"=w356) -> ("States Out"=w357:string)  [unwired: 13 in]
            n89 = Select(t=w357, s=w352, f="") -> (s? t:f=w354:string)
          }
        }
        n90 = Increment(x=w321) -> (x+1=w322:i32)
        n91 = call <vilib>:"Add State(s) to Queue__jki_lib_state_machine.vi"("State(s) in Front (\"\")"=w323, "State(s) in (\"\")"=w335) -> ("States Out"=w336:string)  [unwired: 13 in]
        n92 = call <vilib>:"Add State(s) to Queue__jki_lib_state_machine.vi"("State(s) in (\"\")"=w333) -> ("States Out"=w334:string)  [unwired: 14 in]
      }
      frame "SelectByDatetime" {
        # "Upload"
        n93 = Get Date/Time In Seconds() -> (seconds since 1Jan1904=w374:timestamp)
        n94 = Index Array(array=w362, index #1=14 ("index"), index #2=0 ("index")) -> (element #1=w402:string, element #2=w369:string)
        n95 = Multiply(x=86400.0, y=15.0) -> (x*y=w380:dbl)
        n96 = To Double Precision Float(number=w374) -> (double precision float=w383:dbl)
        n97 = Build Array(w402) -> (w400:string[])
        n98 = Build Array("0" ("State(s) in (\"\")")) -> (w399:string[])
        n99 = Subtract(x=w383, y=w380) -> (x-y=w379:dbl)
        n100 = To Time Stamp(1:w379) -> (0:w375:timestamp)
        n101 = Format Date/Time String(time format string (%c)="%Y-%m-%d ", seconds (now)=w375) -> (date/time string=w378:string)  [unwired: 1 in]
        n102 = Format Date/Time String(time format string (%c)="%Y-%m-%d %H:%M:%S") -> (date/time string=w371:string)  [unwired: 2 in]
        n103 = Concatenate Strings(w378, "00:00:00" ("Numeric Text.Text 2")) -> (w372:string)
        n104 = call <userlib>:"SQL_Select From DB Table.vi"("DB Type"=T4."SQLite", "ColumnsValue"=w399, "ColumnsNameList"=w400, "TableName"=w397) -> ("Select SQL CMD"=w387:string)  [unwired: 7 in]
        n105 = call <userlib>:"Create Between DateTime.vi"("HaveWhere?"=FALSE, "End DateTime"=w371, "Start DateTime"=w372, "Column Name"=w369) -> ("Between DateTime"=w366:string)  [unwired: 7 in]
        n106 = Concatenate Strings(w387, w366) -> (w367:string)
        n107 = call-dynamic "SQL Execute.vi"("error in (no error)"=w392, "Command Text"=w367, "HostDB in"=w396) -> ("error out"=w391:errorcluster, "Table Control"=w365:string[][], "HostDB out"=w395:refnum<class "SQLite.lvclass">)  [unwired: 4 in, 2 out]
        n108 = flat-sequence {
          tunnel: w365 -> [w405]
          tunnel: [w404] -> w364
          frame #0 {
            n109 = for {
              tunnel: w405 -> [w410] mode=indexing
              tunnel: [w409] -> w408 mode=indexing
              n110 = for {
                tunnel: w410 -> [w415] mode=indexing
                tunnel: [w411] -> w409
                i -> [w411]
                stop <- w412 stop-if-true
                n111 = String Length(string=w415) -> (length=w414:i32)
                n112 = Less?(x=w414, y=1) -> (x < y?=w412:bool)
              }
            }
            n113 = Array Max & Min(array=w408) -> (max value=w406:i32)  [unwired: 3 out]
            n114 = Array Subset(array=w405, index (col)=0 ("index"), length (col)=w406) -> (w404:string[][])  [unwired: 2 in]
          }
        }
        n115 = call <vilib>:"Add State(s) to Queue__jki_lib_state_machine.vi"("State(s) in Front (\"\")"=w386, "State(s) in (\"\")"=w367) -> ("States Out"=w388:string)  [unwired: 13 in]
        n116 = Bundle By Name(cluster=w385, "length"=20) -> (w361:T2)
        n117 = call <vilib>:"Add State(s) to Queue__jki_lib_state_machine.vi"("State(s) in (\"\")"=w393) -> ("States Out"=w394:string)  [unwired: 14 in]
        n118 = call <vilib>:"Add State(s) to Queue__jki_lib_state_machine.vi"("State(s) in (\"\")"=w389, "State(s) at Back (\"\")"=w388) -> ("States Out"=w390:string)  [unwired: 13 in]
      }
      frame "Update" {
        n119 = Unbundle By Name(w440) -> ("Row Numbers"=w439:string)
        n120 = Index Array(array=w416, index=1) -> (element=w451:string)
        n121 = Index Array(array=w416, index #1=1 ("index")) -> (element #1=w435:string, element #2=w434:string, element #3=w433:string)  [unwired: 2 in]
        n122 = Build Array("0" ("element"), w447) -> (w430:string[])
        n123 = Build Array(w435, w434, w433) -> (w432:string[])
        n124 = Build Array(w451) -> (w449:string[])
        n125 = Build Array(w439) -> (w438:string[])
        n126 = call <userlib>:"Build string_ColumnsName=ColumnsValue_Where and.vi"("DB Type"=T4."SQLite", "ColumnsValue"=w430, "Check ASCII?"=FALSE, "ColumnsNameList"=w432) -> ("ColumnName='ColumnValue'"=w437:string)  [unwired: 7 in]
        n127 = call <userlib>:"SQL_Update DB Table.vi"("where name='value'"=w437, "ColumnsValue"=w438, "ColumnsNameList"=w449, "TableName"=w448) -> ("Update CMD"=w420:string)  [unwired: 7 in]
        n128 = call-dynamic "SQL Execute.vi"("error in (no error)"=w443, "Return Data (T)"=FALSE, "Command Text"=w420, "HostDB in"=w446) -> ("error out"=w427:errorcluster, "HostDB out"=w445:refnum<class "SQLite.lvclass">)  [unwired: 3 in, 3 out]
        n129 = Select(t="", s=w427, f="Insert") -> (s? t:f=w425:string)
        n130 = call <vilib>:"Add State(s) to Queue__jki_lib_state_machine.vi"("State(s) in Front (\"\")"=w419, "State(s) in (\"\")"=w420) -> ("States Out"=w421:string)  [unwired: 13 in]
        n131 = call <vilib>:"Add State(s) to Queue__jki_lib_state_machine.vi"("State(s) in Front (\"\")"=w425, "State(s) in (\"\")"=w441) -> ("States Out"=w442:string)  [unwired: 13 in]
        n132 = call <vilib>:"Add State(s) to Queue__jki_lib_state_machine.vi"("State(s) in (\"\")"=w422, "State(s) at Back (\"\")"=w421) -> ("States Out"=w423:string)  [unwired: 13 in]
      }
      frame "Update-UploadColumn" {
        n133 = Unbundle By Name(w472) -> ()  [unwired: 1 out]
        n134 = Index Array(array=w453, index=14) -> (element=w483:string)
        "element" <- w483
        n135 = Index Array(array=w453, index #1=1 ("index")) -> (element #1=w468:string, element #2=w467:string)  [unwired: 1 in]
        n136 = Build Array(w455, w479) -> (w465:string[])
        n137 = Build Array(w468, w467) -> (w466:string[])
        n138 = Build Array(w483) -> (w481:string[])
        n139 = Build Array("Upload Num") -> (w471:string[])
        n140 = call <userlib>:"Build string_ColumnsName=ColumnsValue_Where and.vi"("DB Type"=T4."SQLite", "ColumnsValue"=w465, "Check ASCII?"=FALSE, "ColumnsNameList"=w466) -> ("ColumnName='ColumnValue'"=w470:string)  [unwired: 7 in]
        n141 = call <userlib>:"SQL_Update DB Table.vi"("where name='value'"=w470, "ColumnsValue"=w471, "ColumnsNameList"=w481, "TableName"=w480) -> ("Update CMD"=w459:string)  [unwired: 7 in]
        "Update CMD" <- w459
        n142 = call-dynamic "SQL Execute.vi"("error in (no error)"=w475, "Return Data (T)"=FALSE, "Command Text"=w459, "HostDB in"=w478) -> ("HostDB out"=w477:refnum<class "SQLite.lvclass">)  [unwired: 3 in, 4 out]
        n143 = call <vilib>:"Add State(s) to Queue__jki_lib_state_machine.vi"("State(s) in Front (\"\")"=w458, "State(s) in (\"\")"=w459) -> ("States Out"=w460:string)  [unwired: 13 in]
        n144 = call <vilib>:"Add State(s) to Queue__jki_lib_state_machine.vi"("State(s) in (\"\")"=w473) -> ("States Out"=w474:string)  [unwired: 14 in]
        n145 = call <vilib>:"Add State(s) to Queue__jki_lib_state_machine.vi"("State(s) in (\"\")"=w461, "State(s) at Back (\"\")"=w460) -> ("States Out"=w462:string)  [unwired: 13 in]
      }
      frame "Update: FilePath" {
        n146 = Unbundle By Name(w501) -> ("Results Folder path"=w502:path, "RowNum"=w495:i32)  [unwired: 1 out]
        n147 = case shown="2.." w495 {
          selector: w495 -> [_ w532 _]
          tunnel: w504 -> [w530 w535 w537]
          tunnel: [w530 w534 w536] -> w505
          frame Default {
          }
          frame 2.. {
            n148 = Number To Decimal String(number=w532) -> (decimal integer string=w531:string)  [unwired: 1 in]
            n149 = Concatenate Strings(w535, "_" ("string"), w531) -> (w534:string)
          }
          frame 0 {
            n150 = Concatenate Strings(w537) -> (w536:string)
          }
        }
        n151 = call "Get Main.Parmeters.vi"("VariableName"="ResultsFileFormat") -> ("Value"=w491:string)  [unwired: 7 in, 7 out]
        n152 = Empty String/Path?(string/path=w505) -> (empty?=w509:bool)
        n153 = Format Date/Time String(time format string (%c)=w503) -> (date/time string=w508:string)  [unwired: 2 in]
        n154 = Select(t=w508, s=w509, f=w505) -> (s? t:f=w506:string)
        n155 = Concatenate Strings(w506, w491) -> (w507:string)
        n156 = Build Path(base path=w502, name or relative path=w507) -> (appended path=w493:path)
        n157 = Path To String(path=w493) -> (string=w490:string)
        n158 = Index Array(array=w485, index=13) -> (element=w528:string)
        n159 = Index Array(array=w485, index #1=1 ("index")) -> (element #1=w517:string, element #2=w516:string, element #3=w515:string)  [unwired: 2 in]
        n160 = Build Array("0" ("element"), w504) -> (w512:string[])
        n161 = Build Array(w517, w516, w515) -> (w514:string[])
        n162 = Build Array(w528) -> (w526:string[])
        n163 = Build Array(w490) -> (w520:string[])
        n164 = call <userlib>:"Build string_ColumnsName=ColumnsValue_Where and.vi"("DB Type"=T4."SQLite", "ColumnsValue"=w512, "Check ASCII?"=FALSE, "ColumnsNameList"=w514) -> ("ColumnName='ColumnValue'"=w519:string)  [unwired: 7 in]
        n165 = call <userlib>:"SQL_Update DB Table.vi"("where name='value'"=w519, "ColumnsValue"=w520, "ColumnsNameList"=w526, "TableName"=w525) -> ("Update CMD"=w497:string)  [unwired: 7 in]
        n166 = call-dynamic "SQL Execute.vi"("error in (no error)"=w489, "Command Text"=w497, "HostDB in"=w524) -> ("error out"=w487:errorcluster, "HostDB out"=w523:refnum<class "SQLite.lvclass">)  [unwired: 4 in, 3 out]
        n167 = call <vilib>:"Add State(s) to Queue__jki_lib_state_machine.vi"("State(s) in Front (\"\")"=w496, "State(s) in (\"\")"=w497) -> ("States Out"=w498:string)  [unwired: 13 in]
        n168 = Bundle By Name(cluster=w501, "ResultFilePath"=w493) -> (w494:T2)
        n169 = call <vilib>:"Add State(s) to Queue__jki_lib_state_machine.vi"("State(s) in (\"\")"=w499, "State(s) at Back (\"\")"=w498) -> ("States Out"=w500:string)  [unwired: 13 in]
        n170 = call <vilib>:"Add State(s) to Queue__jki_lib_state_machine.vi"("State(s) in (\"\")"=w521) -> ("States Out"=w522:string)  [unwired: 14 in]
      }
      frame "Close" {
        n171 = call-dynamic "Close Connection.vi"("error in (no error)"=w539, "HostDB in"=w541) -> ("error out"=w538:errorcluster, "HostDB out"=w540:refnum<class "SQLite.lvclass">)  [unwired: 8 in]
      }
    }
  }
  "CMD" <- w17
  n172 = Random Number (0-1)() -> (number: 0 to 1=→"number (0 to 1)":dbl)
  n173 = Unbundle By Name(w3) -> ("length"=w2:i32)
  n174 = disable-structure shown="Disabled" {
    disable-tunnel: w13 -> [w549 _]
    frame Disabled {
      "Table Control" <- w549
    }
    frame Enabled {
    }
  }
  n175 = Merge Errors(w22) -> (→"error out":errorcluster)
  n176 = Array Subset(array=w13, index (row)=0 ("index"), length (row)=w2) -> (w9:string[][])  [unwired: 2 in]
  n177 = Index Array(array=w9, index (col)=13 ("disabled index (col)")) -> (element=→"File Paht":string[])  [unwired: 1 in]
  n178 = Delete From Array(array=w9, length=1, index (col)=0 ("disabled index (col)")) -> (array with subset deleted=→"30 rows":string[][])  [unwired: 1 in, 1 out]
